vi "LOGIC_toLogical.vi"(7 "error in (no error)":errorcluster, 9 "command":string) -> (0 "error out":errorcluster)   [LabVIEW 2016]
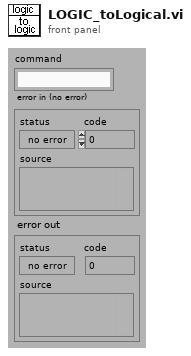
[diagram p1: front panel]
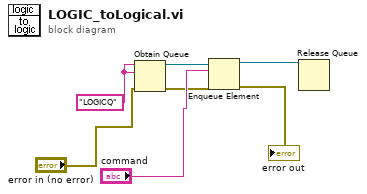
[diagram p0: block diagram]
diagram:
  w1 = "LOGICQ" ("name (unnamed)")
  n1 = Obtain Queue(name (unnamed)=w1, element data type=w1, error in (no error)="error in (no error)") -> (queue out=w7:refnum<queue>, error out=w4:errorcluster)  [unwired: 2 in, 1 out]
  n2 = Enqueue Element(queue=w7, element="command", error in (no error)=w4) -> (queue out=w2:refnum<queue>, error out=→"error out":errorcluster)  [unwired: 2 out]
  n3 = Release Queue(queue=w2) -> ()  [unwired: 1 in, 4 out]
